vi "Class Generator.vi"(0 "#":u32) -> (1 "psi":i32[](array[numeric]), 2 "psi^-1":i32[](array[numeric]), 3 "prime":bool)   [LabVIEW 2024, in "NI_Gmath.lvlib"]
uses:
  NI_Gmath.lvlib
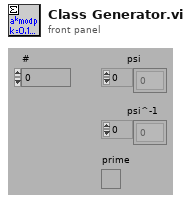
[diagram p1: front panel]
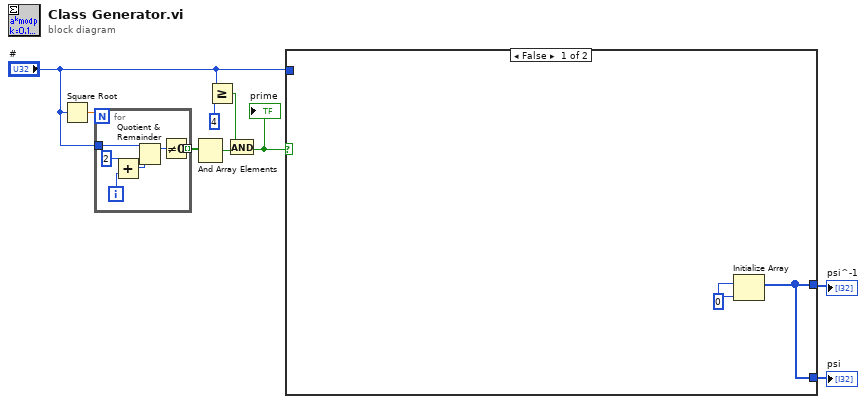
[diagram p0: block diagram]
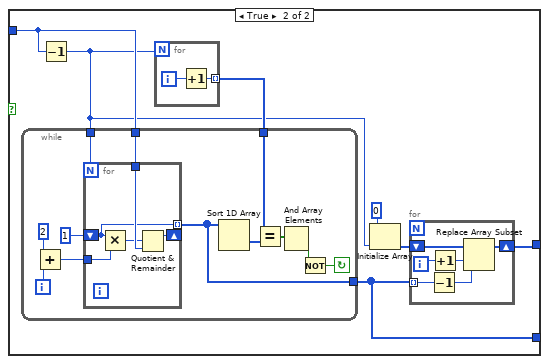
[diagram p2: hidden frame]
diagram:
  n1 = Square Root(x="#") -> (sqrt(x)=w9:dbl)
  n2 = for {
    N: w9 -> [_]
    tunnel: "#" -> [w15]
    tunnel: [w10] -> w8 mode=indexing
    i -> [w13]
    n3 = Add(x=2, y=w13) -> (x+y=w12:i32)
    n4 = Quotient & Remainder(x=w15, y=w12) -> (x-y*floor(x/y)=w11:u32)  [unwired: 1 out]
    n5 = Not Equal To 0?(x=w11) -> (x != 0?=w10:bool)
  }
  n6 = And Array Elements(Boolean array=w8) -> (logical AND=w5:bool)
  n7 = Greater Or Equal?(x="#", y=4) -> (x >= y?=w4:bool)
  n8 = And(x=w4, y=w5) -> (x .and. y?=w3:bool)
  "prime" <- w3
  n9 = case shown="False" w3 {
    tunnel: "#" -> [_ w22]
    tunnel: [w16 w19] -> w7
    tunnel: [w16 w18] -> w6
    frame False {
      w17 = 0
      n10 = Initialize Array(w17, w17) -> (w16:i32[])
    }
    frame True {
      n11 = Decrement(x=w22) -> (x-1=w20:u32)
      n12 = for {
        N: w20 -> [_]
        tunnel: [w42] -> w21 mode=indexing
        i -> [w43]
        n13 = Increment(x=w43) -> (x+1=w42:i32)
      }
      n14 = while {
        tunnel: [w25] -> w18
        tunnel: w21 -> [w30]
        tunnel: w20 -> [w31]
        tunnel: w22 -> [w32]
        i -> [w36]
        stop <- w27 continue-if-true
        n15 = Add(x=2, y=w36) -> (x+y=w33:i32)
        n16 = for {
          N: w31 -> [_]
          shift-right: [w38] -> _
          shift-left: 1 -> [w37]
          tunnel: w33 -> [w41]
          tunnel: w32 -> [w40]
          tunnel: [w37] -> w25 mode=indexing
          n17 = Multiply(x=w37, y=w41) -> (x*y=w39:u32)
          n18 = Quotient & Remainder(x=w39, y=w40) -> (x-y*floor(x/y)=w38:u32)  [unwired: 1 out]
        }
        n19 = Sort 1D Array(array=w25) -> (sorted array=w26:u32[])
        n20 = Equal?(x=w30, y=w26) -> (x = y?=w29:bool[])
        n21 = And Array Elements(Boolean array=w29) -> (logical AND=w28:bool)
        n22 = Not(x=w28) -> (.not. x?=w27:bool)
      }
      n23 = Initialize Array(0, w20) -> (w24:i32[])
      n24 = for {
        shift-right: [w48] -> w19
        shift-left: w24 -> [w49]
        tunnel: w18 -> [w45] mode=indexing
        i -> [w47]
        n25 = Decrement(x=w45) -> (x-1=w44:u32)
        n26 = Increment(x=w47) -> (x+1=w46:i32)
        n27 = Replace Array Subset(array=w49, new element=w46, index=w44) -> (w48:i32[])
      }
    }
  }
  "psi" <- w6
  "psi^-1" <- w7
